vi "POST_changeServoStatus.vi"(3 "LabVIEW Web Service Request":refnum<class "Web Request.lvclass">) -> (1 "response":string)   [LabVIEW 2024]
uses:
  <vilib>/wsapi/Web Request.lvclass
panel:
  out "Status From Client":cluster{"mode":string, "position":dbl}
  # "Use the Web Service Request input terminal to call the VIs on the Web Services palette. Do not remove it from the connector pane unless you don't need access to the palette."
  # "Each additional control wired to the connector pane will be available as an input in the URL. To include an indicator in terminal-mode output (the default setting), it must also be wired to the connector pane."
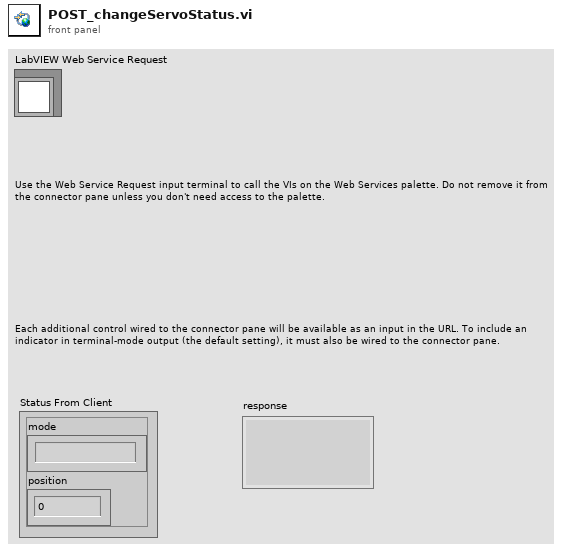
[diagram p1: front panel]
types:
  T1 = cluster{"status":cluster{"mode":string, "position":dbl}}
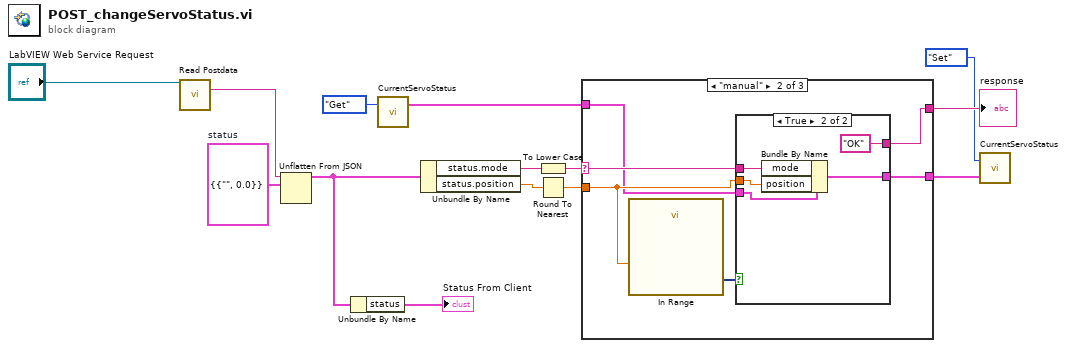
[diagram p0: block diagram]
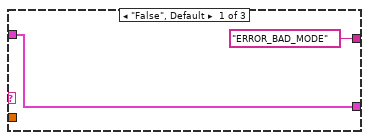
[diagram p2: hidden frame]
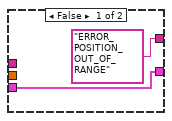
[diagram p3: hidden frame]
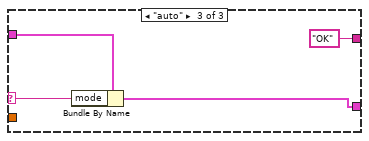
[diagram p4: hidden frame]
diagram:
  w7 = T1 {"status"={"mode"="", "position"=0.0}}  # status
  n1 = call <vilib>:"Read Postdata.vi"("LabVIEW Web Service Request"="LabVIEW Web Service Request") -> ("postdata"=w13:string)  [unwired: 12 in, 2 out]
  n2 = Unflatten From JSON(JSON string=w13, type and defaults=w7) -> (value=w2:T1)  [unwired: 5 in, 1 out]
  n3 = Unbundle By Name(w2) -> ("status"=→"Status From Client":cluster{"mode":string, "position":dbl})
  n4 = call "CurrentServoStatus.vi"("Operation"=enum16{"Get", "Set", ""}."Get") -> ("Current Servo Status"=w6:cluster{"mode":string, "position":dbl})  [unwired: 2 in]
  n5 = Unbundle By Name "Unbundle By Name"(w2) -> ("status.mode"=w11:string, "status.position"=w12:dbl)
  n6 = To Lower Case(string=w11) -> (all lower case string=w9:string)
  n7 = Round To Nearest(number=w12) -> (nearest integer value=w8:dbl)
  n8 = case shown="\"manual\"" w9 {
    selector: w9 -> [_ w19 w32]
    tunnel: w8 -> [_ w20 _]
    tunnel: ["ERROR_BAD_MODE" w21 "OK"] -> w10
    tunnel: w6 -> [w15 w17 w30]
    tunnel: [w15 w18 w31] -> w3
    frame "False", Default {
    }
    frame "manual" {
      n9 = call "In Range"("Operand 1"=w20) -> ("Result"=w22:dynamicdata)  [unwired: 9 in, 1 out]
      n10 = case shown="True" w22 {
        tunnel: ["ERROR_POSITION_OUT_OF_RANGE" "OK"] -> w21
        tunnel: w20 -> [_ w26]
        tunnel: w19 -> [_ w27]
        tunnel: w17 -> [w23 w28]
        tunnel: [w23 w25] -> w18
        frame False {
        }
        frame True {
          n11 = Bundle By Name(cluster=w28, "mode"=w27, "position"=w26) -> (w25:cluster{"mode":string, "position":dbl})
        }
      }
    }
    frame "auto" {
      n12 = Bundle By Name(cluster=w30, "mode"=w32) -> (w31:cluster{"mode":string, "position":dbl})
    }
  }
  "response" <- w10
  n13 = call "CurrentServoStatus.vi"("New Servo Status"=w3, "Operation"=enum16{"Get", "Set", ""}."Set") -> ()  [unwired: 1 in, 1 out]
